vi "GetState.vi"(0 "reference in":refnum<class "mmWave instrument.lvclass">, 11 "error in (no error)":errorcluster) -> (4 "reference out":refnum<class "mmWave instrument.lvclass">, 6 "state":T2, 8 "mode":T1, 10 "state (str)":string, 15 "error out":errorcluster)   [LabVIEW 2019, in "mmWave instrument.lvclass"]
doc: "Returns active state of instrument"
uses:
  mmWave instrument.lvclass
  Instrument state.ctl
  Instrument mode.ctl
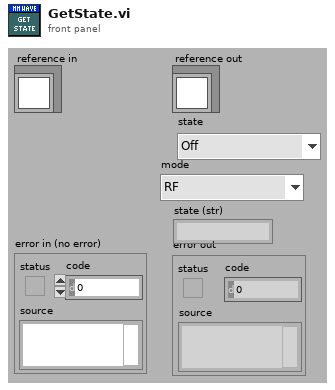
[diagram p1: front panel]
types:
  T1 = typedef "mmWave instrument.lvclass/Instrument mode.ctl" = enum16{"RF", "IF", "BB"}
  T2 = typedef "mmWave instrument.lvclass/Instrument state.ctl" = enum16{"Off", "Initialization", "Configuration", "Running", "Calibration"}
  T3 = typedef "mmWave instrument.lvclass/ObjectAttributes.ctl" = cluster{"mode":T1, "instr state":T2, "Max Fs":dbl, "Equalization coeff":cdb[], "LO sync en":bool, "Trig sync en":bool, "LO sources":T4, "LO Export":T5, "Fc.range":cluster{"min":dbl, "max":dbl}, "Sync mode":T6, "equalization en":bool, "sequence":string[]}
  T4 = typedef "mmWave HW Control.lvlib/LO sources.ctl" = cluster{"RX/LO1 src":string, "TX/LO1 src":string, "LO2 src":string}
  T5 = typedef "mmWave HW Control.lvlib/LO export.ctl" = cluster{"TX LO1 export":bool, "TX LO1 export level":dbl, "RX LO1 export":bool, "RX LO1 export level":dbl, "LO2 export":bool, "LO2 export level":dbl}
  T6 = typedef "mmWave instrument.lvclass/Sync mode.ctl" = enum16{"Slave", "Master"}
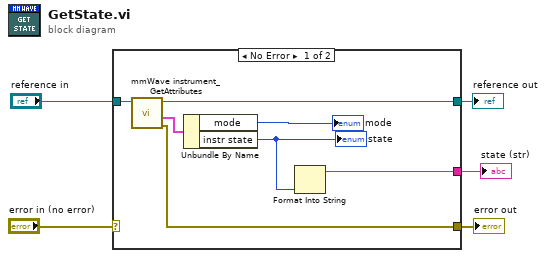
[diagram p0: block diagram]
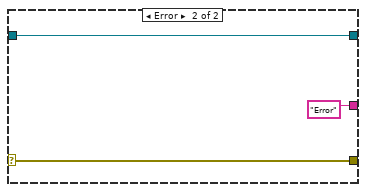
[diagram p2: hidden frame]
diagram:
  n1 = case shown="No Error" "error in (no error)" {
    selector: "error in (no error)" -> [_ w15]
    tunnel: [w12 w15] -> w4
    tunnel: [w11 w14] -> w2
    tunnel: "reference in" -> [w9 w14]
    tunnel: [w7 "Error"] -> w1
    frame No Error {
      n2 = call "mmWave instrument_GetAttributes.vi"("reference in"=w9) -> ("error out"=w12:errorcluster, "attributes"=w10:T3, "reference out"=w11:refnum<class "mmWave instrument.lvclass">)  [unwired: 7 in, 1 out]
      n3 = Unbundle By Name(w10) -> ("mode"=→"mode":T1, "instr state"=w8:T2)
      "state" <- w8
      n4 = Format Into String(w8) -> (resulting string=w7:string)  [unwired: 3 in, 1 out]
    }
    frame Error {
    }
  }
  "error out" <- w4
  "reference out" <- w2
  "state (str)" <- w1
